vi "SVPO Limit Testing (Scalar) (DBL).vi"(7 "reset? (F)":bool, 9 "lower limit":dbl=-inf format="%.2f", 10 "upper limit":dbl=inf format="%.2f", 11 "value in":dbl=inf format="%.2f") -> (1 "lower limit clearance":dbl format="%.6f", 2 "upper limit clearance":dbl format="%.6f", 3 "test passed?":bool)   [LabVIEW 2017, in "SoundVib_LimitTest.lvlib"]
doc: "Performs limit testing on single-precision waveforms, single-precision scaled arrays, or double-precision scalar measurements. You can specify an upper and lower boundary of the envelope to define a pass range. This VI uses the defined pass range to test the input signal. VI outputs apply to all the tests since the last VI reset. Use this VI on embedded targets that have limited computational resources. Wire data to the <B>value in</B> input to determine the polymorphic instance to use or manually select the instance."
uses:
  <vilib>/addons/Sound and Vibration/svt_Limit Test/SoundVib_LimitTest.lvlib
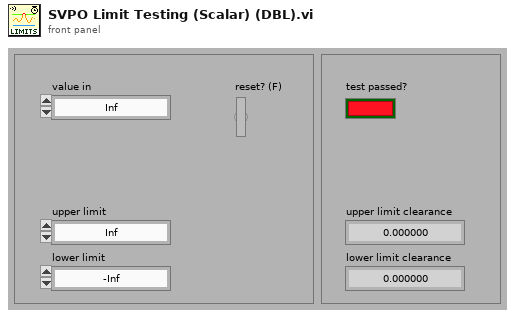
[diagram p1: front panel]
types:
  T1 = typedef "svc_DBL Limit State.ctl" = cluster{"upper limit clearance":dbl, "lower limit clearance":dbl, "test passed?":bool}
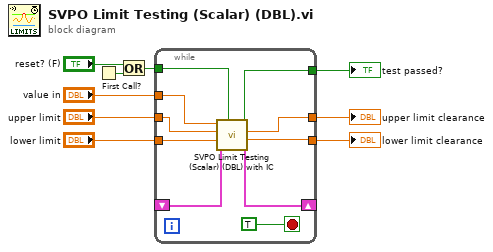
[diagram p0: block diagram]
diagram:
  n1 = First Call?() -> (First Call?: T/F=w5:bool)
  n2 = Or(x="reset? (F)", y=w5) -> (x .or. y?=w6:bool)
  n3 = while {
    tunnel: "value in" -> [w17]
    tunnel: "upper limit" -> [w16]
    tunnel: "lower limit" -> [w15]
    tunnel: w6 -> [w18]
    shift-right: [w14] -> _
    shift-left: _ -> [w13]
    tunnel: [w12] -> w3
    tunnel: [w11] -> w2
    tunnel: [w10] -> w1
    stop <- TRUE stop-if-true
    n4 = call <vilib>:"SVPO Limit Testing (Scalar) (DBL) with IC.vi"("reset? (F)"=w18, "initial conditions"=w13, "lower limit"=w15, "upper limit"=w16, "value in"=w17) -> ("final conditions"=w14:T1, "lower limit clearance"=w11:dbl, "upper limit clearance"=w10:dbl, "test passed?"=w12:bool)  [unwired: 3 in]
  }
  "test passed?" <- w3
  "upper limit clearance" <- w1
  "lower limit clearance" <- w2
